vi "LEBITplc.destructor.vi"(0 "i ref in":refnum<vi>, 5 "error in(no error)":errorcluster) -> (19 "error out":errorcluster)   [LabVIEW 2014, in "LEBITplc.lvlib"]
doc: "This is the destructor of a class.\n\nLicense Agreement for this software:\n\nCopyright (C)\nGesellschaft für Schwerionenforschung, GSI\nPlanckstr. 1\n64291 Darmstadt\nGermany\n\nContact: D.Beck@gsi.de \n\nThis program is free software; you can redistribute it and/or modify it under the terms of the \nGNU General Public License as published by the Free Software Foundation; either version 2 of \nthe license, or (at your option) any later version.\n\nThis program is distributed in the hope that it will be useful, but WITHOUT ANY WARRANTY; \nwithout even the implied warranty of MERCHANTABILITY or FITNESS FOR A PARTICULAR PURPOSE. See the GNU General License for more details (http://www.gnu.org).\n\nGesellschaft für Schwerionenforschung, GSI\nPlanckstr. 1, 64291 Darmstadt, Germany\nFor all questions and ideas contact: M.Richter@gsi.de, H.Brand@gsi.de or D.Beck@gsi.de.\nLast update: 16-JUN-2004"
uses:
  LEBITplc.lvlib
  CSCore/BaseProcess/BaseProcess.lvlib
  CSlibraries-extern/DimLVEvent/LVDimInterface/LVDimInterface.lvlib
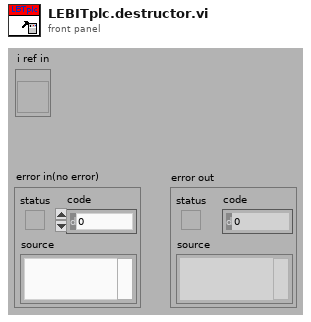
[diagram p1: front panel]
types:
  T1 = typedef "LEBITplc.lvlib/LEBITplc.i attribute.ctl" = cluster{"LLFLocation":string, "SetFileLocation":string, "nickNames":string[], "setValuePLCServiceID":i32[], "GUIServiceID":i32[], "monValuePLC":string[], "SetValueServiceID":i32[], "MonValueServiceID":i32[], "SetValue":dbl[][], "SetValueMin":dbl[], "SetValueMax":dbl[], "SetValueInfoServiceID":i32[], "GUINames":string[], "ListOfBases":string[], "Scale":dbl[], "Offset":dbl[], "setValuePLC":string[], "BaseName":string[], "ScaleServiceID":i32[], "OffsetServiceID":i32[], "AllPLCValues":string[], "CondSpecialArray":string[][], "CondSpecialIndex":i32[], "CondSpecialMonValue":dbl[], "RecentlyChanged":i32[], "SetFileLocationID":i32, "Dependent-Monitors":string[][], "LastLoadedFiles":string[], "IonGuideCalibLocation":string, "Monitor Dependent":string[], "Special":string[], "PLC?":bool[], "Start Date":string, "ListOfBasesServiceID":i32, "SETRA VISA resource":refnum<visa-resource-name>}
  T2 = enum16{"SetAttribute", "GetAttribute", "CreateAttribute", "DestroyAttribute", "DestroyAllAtributes"}
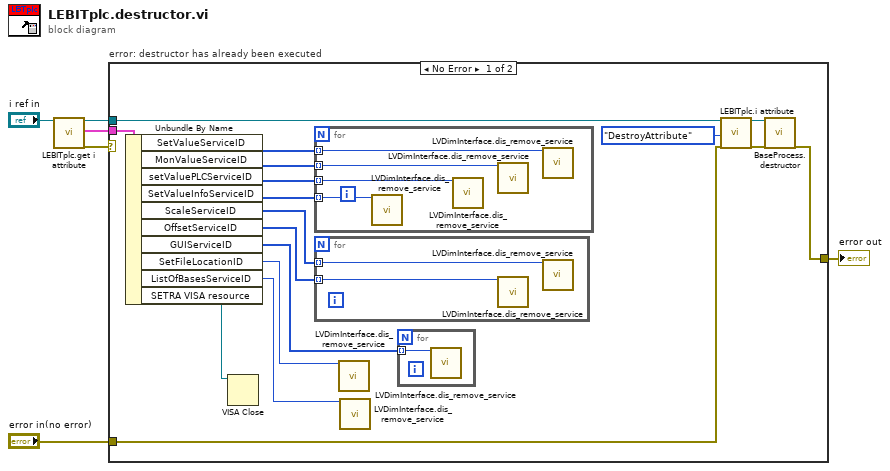
[diagram p0: block diagram]
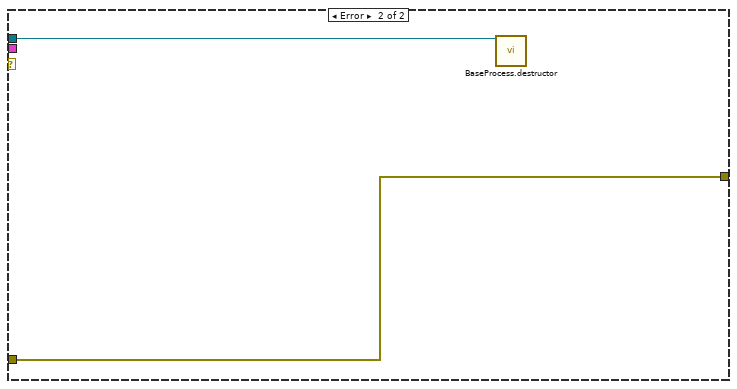
[diagram p2: hidden frame]
diagram:
  n1 = call "LEBITplc.get i attribute.vi"("i ref in"="i ref in") -> ("i ref out"=w2:refnum<vi>, "i attribute"=w1:T1, "error out"=w3:errorcluster)  [unwired: 16 in]
  n2 = case "error: destructor has already been executed" shown="No Error" w3 {
    tunnel: [w14 w32] -> w6
    tunnel: "error in(no error)" -> [w11 w32]
    tunnel: w2 -> [w20 w31]
    tunnel: w1 -> [w19 _]
    frame No Error {
      n3 = Unbundle By Name(w19) -> ("SetValueServiceID"=w18:i32[], "MonValueServiceID"=w17:i32[], "setValuePLCServiceID"=w16:i32[], "SetValueInfoServiceID"=w15:i32[], "ScaleServiceID"=w13:i32[], "OffsetServiceID"=w12:i32[], "GUIServiceID"=w9:i32[], "SetFileLocationID"=w10:i32, "ListOfBasesServiceID"=w8:i32, "SETRA VISA resource"=w7:refnum<visa-resource-name>)
      n4 = VISA Close(VISA resource name=w7) -> ()  [unwired: 1 in, 1 out]
      n5 = for {
        tunnel: w18 -> [w30] mode=indexing
        tunnel: w17 -> [w29] mode=indexing
        tunnel: w16 -> [w28] mode=indexing
        tunnel: w15 -> [w27] mode=indexing
        n6 = call "LVDimInterface.dis_remove_service.vi"("my_serviceID"=w27) -> ()  [unwired: 18 in, 1 out]
        n7 = call "LVDimInterface.dis_remove_service.vi"("my_serviceID"=w28) -> ()  [unwired: 18 in, 1 out]
        n8 = call "LVDimInterface.dis_remove_service.vi"("my_serviceID"=w29) -> ()  [unwired: 18 in, 1 out]
        n9 = call "LVDimInterface.dis_remove_service.vi"("my_serviceID"=w30) -> ()  [unwired: 18 in, 1 out]
      }
      n10 = for {
        tunnel: w13 -> [w26] mode=indexing
        tunnel: w12 -> [w25] mode=indexing
        n11 = call "LVDimInterface.dis_remove_service.vi"("my_serviceID"=w25) -> ()  [unwired: 18 in, 1 out]
        n12 = call "LVDimInterface.dis_remove_service.vi"("my_serviceID"=w26) -> ()  [unwired: 18 in, 1 out]
      }
      n13 = call "LVDimInterface.dis_remove_service.vi"("my_serviceID"=w10) -> ()  [unwired: 18 in, 1 out]
      n14 = call "LVDimInterface.dis_remove_service.vi"("my_serviceID"=w8) -> ()  [unwired: 18 in, 1 out]
      n15 = for {
        tunnel: w9 -> [w24] mode=indexing
        n16 = call "LVDimInterface.dis_remove_service.vi"("my_serviceID"=w24) -> ()  [unwired: 18 in, 1 out]
      }
      n17 = call "LEBITplc.i attribute.vi"("VI Refnum"=w20, "Action"=T2."DestroyAttribute", "error in (no error)"=w11) -> ("VI Refnum out"=w22:refnum<vi>, "error out"=w21:errorcluster)  [unwired: 14 in, 1 out]
      n18 = call "BaseProcess.destructor.vi"("i ref in"=w22, "error in (no error)"=w21) -> ("error out"=w14:errorcluster)  [unwired: 17 in]
    }
    frame Error {
      n19 = call "BaseProcess.destructor.vi"("i ref in"=w31) -> ()  [unwired: 18 in, 1 out]
    }
  }
  "error out" <- w6
